vi "DiffDrivePoseEst2_Update.vi"(6 "Time":dbl=-1.0 format="%33.4f", 8 "RightDistance":dbl, 9 "LeftDistance":dbl, 10 "GyroAngle":T3={"VALUE"=0.0, "COS"=1.0, "SIN"=0.0} {"SIN" format="%13.4f"; "COS" format="%13.4f"; "VALUE" format="%13.4f"}, 11 "in DiffDrivePoseEstimate":T4={"M_Vision_K"=[], "m_nominal_dT"=0.0, "m_PrevTime_Sec"=0.0, "Pose_Buffer"={"TimeStamps"=[], "DataArray"=[], "Min_TimeStamp"=0.0, "Max_TimeStamp"=0.0, "ItemCount"=0, "MaxBufferTime"=0.0}, "Diff_Drive_Kinematics"={"TrackWidth_Meters"=0.0}, "Diff_Drive_Odom_2"={"M_POSE_Meters"={"TRANSLATION"={"X"=0.0, "Y"=0.0}, "ROTATION"={"VALUE"=0.0, "COS"=1.0, "SIN"=0.0}}, "M_GyroOffset"={"VALUE"=0.0, "COS"=1.0, "SIN"=0.0}, "M_PrevAngle"={"VALUE"=0.0, "COS"=1.0, "SIN"=0.0}, "M_PrevLeftDist_M"=0.0, "M_PrevRightDist_M"=0.0, "M_InitLeftDist_M"=0.0, "M_InitRightDist_M"=0.0}, "M_Q"=[[0.0], [0.0], [0.0]]} {"Diff_Drive_Odom_2"."M_PrevAngle"."SIN" format="%13.4f"; "Diff_Drive_Odom_2"."M_PrevAngle"."COS" format="%13.4f"; "Diff_Drive_Odom_2"."M_PrevAngle"."VALUE" format="%13.4f"; "Diff_Drive_Odom_2"."M_GyroOffset"."SIN" format="%13.4f"; "Diff_Drive_Odom_2"."M_GyroOffset"."COS" format="%13.4f"; "Diff_Drive_Odom_2"."M_GyroOffset"."VALUE" format="%13.4f"; "Diff_Drive_Odom_2"."M_POSE_Meters"."ROTATION"."SIN" format="%13.4f"; "Diff_Drive_Odom_2"."M_POSE_Meters"."ROTATION"."COS" format="%13.4f"; "Diff_Drive_Odom_2"."M_POSE_Meters"."ROTATION"."VALUE" format="%13.4f"; "Diff_Drive_Odom_2"."M_POSE_Meters"."TRANSLATION"."Y" format="%14.3f"; "Diff_Drive_Odom_2"."M_POSE_Meters"."TRANSLATION"."X" format="%14.3f"; "Diff_Drive_Kinematics"."TrackWidth_Meters" format="%20.4f"}) -> (0 "Error":bool, 2 "Estimated Pose":T1 {"ROTATION"."SIN" format="%13.4f"; "ROTATION"."COS" format="%13.4f"; "ROTATION"."VALUE" format="%13.4f"; "TRANSLATION"."Y" format="%14.3f"; "TRANSLATION"."X" format="%14.3f"}, 3 "Out DiffDrivePoseEstimate":T4={"M_Vision_K"=[], "m_nominal_dT"=0.0, "m_PrevTime_Sec"=0.0, "Pose_Buffer"={"TimeStamps"=[], "DataArray"=[], "Min_TimeStamp"=0.0, "Max_TimeStamp"=0.0, "ItemCount"=0, "MaxBufferTime"=0.0}, "Diff_Drive_Kinematics"={"TrackWidth_Meters"=0.0}, "Diff_Drive_Odom_2"={"M_POSE_Meters"={"TRANSLATION"={"X"=0.0, "Y"=0.0}, "ROTATION"={"VALUE"=0.0, "COS"=1.0, "SIN"=0.0}}, "M_GyroOffset"={"VALUE"=0.0, "COS"=1.0, "SIN"=0.0}, "M_PrevAngle"={"VALUE"=0.0, "COS"=1.0, "SIN"=0.0}, "M_PrevLeftDist_M"=0.0, "M_PrevRightDist_M"=0.0, "M_InitLeftDist_M"=0.0, "M_InitRightDist_M"=0.0}, "M_Q"=[[0.0], [0.0], [0.0]]} {"Diff_Drive_Odom_2"."M_PrevAngle"."SIN" format="%13.4f"; "Diff_Drive_Odom_2"."M_PrevAngle"."COS" format="%13.4f"; "Diff_Drive_Odom_2"."M_PrevAngle"."VALUE" format="%13.4f"; "Diff_Drive_Odom_2"."M_GyroOffset"."SIN" format="%13.4f"; "Diff_Drive_Odom_2"."M_GyroOffset"."COS" format="%13.4f"; "Diff_Drive_Odom_2"."M_GyroOffset"."VALUE" format="%13.4f"; "Diff_Drive_Odom_2"."M_POSE_Meters"."ROTATION"."SIN" format="%13.4f"; "Diff_Drive_Odom_2"."M_POSE_Meters"."ROTATION"."COS" format="%13.4f"; "Diff_Drive_Odom_2"."M_POSE_Meters"."ROTATION"."VALUE" format="%13.4f"; "Diff_Drive_Odom_2"."M_POSE_Meters"."TRANSLATION"."Y" format="%14.3f"; "Diff_Drive_Odom_2"."M_POSE_Meters"."TRANSLATION"."X" format="%14.3f"; "Diff_Drive_Kinematics"."TrackWidth_Meters" format="%20.4f"})   [LabVIEW 2019, in "Trajectory_Library.lvlib"]
doc: "Updates the the Unscented Kalman Filter using only wheel encoder information. Note that this should be called every loop.\n\nInputs:\n - LeftSpeed -- Left wheel speed (meters/sec)\n - RightSpeed -- Right wheel speed (meters/sec)\n - inDiffDrivePoseEst -- system data cluster\n - gyroAngle -- The current gyro angle. (radians)\n - distanceLeftMeters -- The total distance travelled by the left wheel in meters. This can be the encoder reading.\n - distanceRightMeters -- The total distance travelled by the right wheel in meters. This can be the encoder reading.\n\nOutputs:\n - outDiffDrivePoseEst -- system data cluster\n - EstimatedPose -- The estimated pose of the robot in meters."
uses:
  Trajectory_Library.lvlib
  <vilib>/Analysis/Matrix/Datatypes/RealMatrix.ctl
  <vilib>/Analysis/Matrix/NI_Matrix.lvlib
  TypeDef/ROTATION2D.ctl
  TypeDef/TRANSLATION2D.ctl
  TypeDef/POSE2D.ctl
  TypeDef/TIME_INTERPOLATABLE_VARIANT.ctl
  TypeDef/DIFF_DRIVE_KINEMATICS.ctl
  TypeDef/DIFF_DRIVE_ODOM2.ctl
  TypeDef/DIFF_DRIVE_POSE_EST2.ctl
panel:
  # "<3, 1>"
  # "<3, 3>"
  # "<3, 1>"
  # "<3, 3>"
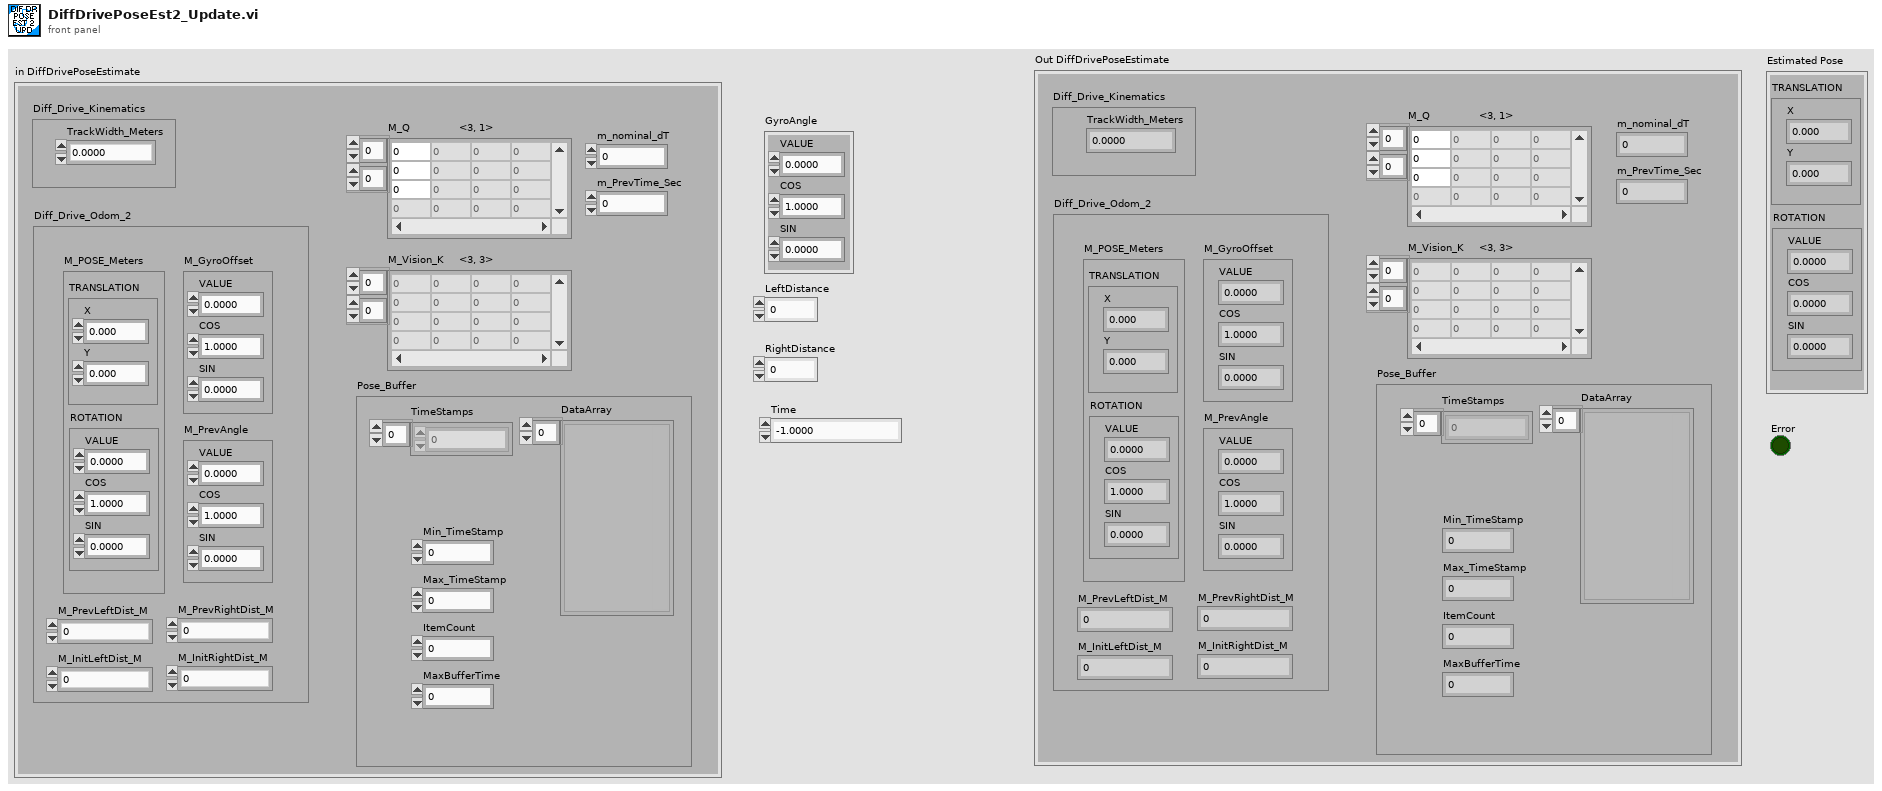
[diagram p1: front panel]
types:
  T1 = typedef "Trajectory_Library.lvlib/POSE2D.ctl" = cluster{"TRANSLATION":T2, "ROTATION":T3}
  T2 = typedef "Trajectory_Library.lvlib/TRANSLATION2D.ctl" = cluster{"X":dbl, "Y":dbl}
  T3 = typedef "Trajectory_Library.lvlib/ROTATION2D.ctl" = cluster{"VALUE":dbl, "COS":dbl, "SIN":dbl}
  T4 = typedef "Trajectory_Library.lvlib/DIFF_DRIVE_POSE_EST2.ctl" = cluster{"M_Vision_K":T5, "m_nominal_dT":dbl, "m_PrevTime_Sec":dbl, "Pose_Buffer":T6, "Diff_Drive_Kinematics":T7, "Diff_Drive_Odom_2":T8, "M_Q":T5}
  T5 = typedef "NI_Matrix.lvlib/RealMatrix.ctl" = dbl[][]
  T6 = typedef "Trajectory_Library.lvlib/TIME_INTERPOLATABLE_VARIANT.ctl" = cluster{"TimeStamps":dbl[], "DataArray":variant[], "Min_TimeStamp":dbl, "Max_TimeStamp":dbl, "ItemCount":i32, "MaxBufferTime":dbl}
  T7 = typedef "Trajectory_Library.lvlib/DIFF_DRIVE_KINEMATICS.ctl" = cluster{"TrackWidth_Meters":dbl}
  T8 = typedef "Trajectory_Library.lvlib/DIFF_DRIVE_ODOM2.ctl" = cluster{"M_POSE_Meters":T1, "M_GyroOffset":T3, "M_PrevAngle":T3, "M_PrevLeftDist_M":dbl, "M_PrevRightDist_M":dbl, "M_InitLeftDist_M":dbl, "M_InitRightDist_M":dbl}
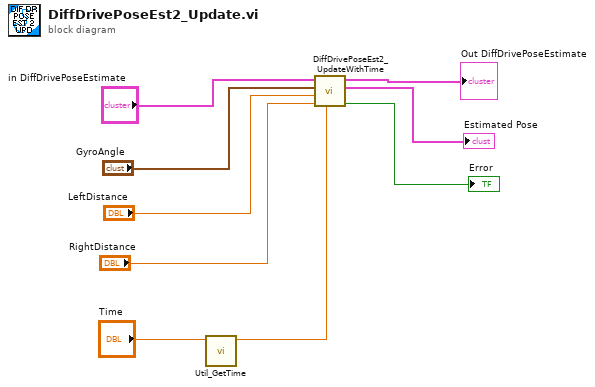
[diagram p0: block diagram]
diagram:
  n1 = call "Util_GetTime.vi"("Pass_Through_Time"="Time") -> ("FPGA_Time_Seconds"=w1:dbl)  [unwired: 8 in, 2 out]
  n2 = call "DiffDrivePoseEst2_UpdateWithTime.vi"("CurrentTimeSeconds"=w1, "RightDistance"="RightDistance", "LeftDistance"="LeftDistance", "GyroAngle"="GyroAngle", "in DiffDrivePoseEstimate"="in DiffDrivePoseEstimate") -> ("Error"=→"Error":bool, "Estimated Pose"=→"Estimated Pose":T1, "Out DiffDrivePoseEstimate"=→"Out DiffDrivePoseEstimate":T4)  [unwired: 4 in]
